vi "Worker lvlib Icon.vi"(9 "Icon Active":bool, 11 "Item Ref In":T1) -> (3 "Item Ref":T1)   [LabVIEW 2020, in "FlexWorker_Provider.lvlib"]
uses:
  FlexWorker_Provider.lvlib
  <resource>/Framework/Providers/API/ItemRef.ctl
  <resource>/Framework/Providers/API/mxLvUpdateUI.ctl
  <resource>/Framework/Providers/API/mxLvOverlayState.ctl
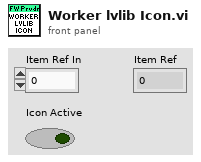
[diagram p1: front panel]
types:
  T1 = typedef "ItemRef.ctl" = u64
  T2 = typedef "mxLvOverlayState.ctl" = cluster{"Overlay Alias":string, "Active":bool}
  T3 = typedef "mxLvUpdateUI.ctl" = cluster{"Action":u32, "Optional param 1":string, "Optional param 2":i32, "Optional param 3":string}
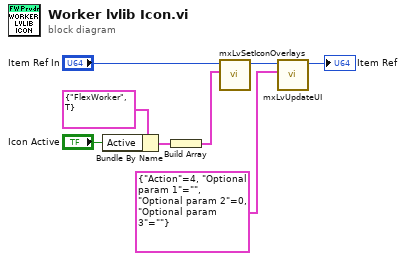
[diagram p0: block diagram]
diagram:
  n1 = Bundle By Name(cluster=T2 {"Overlay Alias"="FlexWorker", "Active"=TRUE} ("Icon Overlay State"), "Active"="Icon Active") -> (w5:T2)
  n2 = Build Array(w5) -> (w4:T2[])
  n3 = call <resource>:"mxLvSetIconOverlays.vi"("Overlay States"=w4, "Item"="Item Ref In") -> ("Item"=w8:T1)  [unwired: 8 in, 1 out]
  n4 = call <resource>:"mxLvUpdateUI.vi"("Update UI Settings"=T3 {"Action"=4, "Optional param 1"="", "Optional param 2"=0, "Optional param 3"=""}, "Item"=w8) -> ("Item"=→"Item Ref":T1)  [unwired: 8 in, 1 out]
